vi "FetchRX.vi"(8 "error in (no error)":errorcluster, 11 "reference in":refnum<class "niMmWave_Transceiver.lvclass">) -> (0 "error out":errorcluster, 2 "RX burst data":refnum<class "mmWave data.lvclass">, 3 "reference out":refnum<class "niMmWave_Transceiver.lvclass">)   [LabVIEW 2019, in "niMmWave_Transceiver.lvclass"]
doc: "Fetches RX IQ data from isnturment"
uses:
  niMmWave_Transceiver.lvclass
  C:/Barkhausen mmWave radar/Development/modules/mmw_instrument/src_LabVIEW/Host/SubVIs/mmWave instrument_class/mmWave instrument.lvclass
  mmWave data_class/mmWave data.lvclass
  mmWave HW Control/HW custom error.ctl
  IQBurst_memo_class/IQBurst_memo.lvclass
  C:/Barkhausen mmWave radar/Development/modules/mmw_instrument/src_LabVIEW/Host/SubVIs/mmWave data_class/mmWave data.lvclass
  mmWave instrument_class/Instrument state.ctl
  032ac389-5447-437e-ad81-02506a350dfa.vi
  <vilib>/addons/Modulation/Analog/MT Resample (Complex Cluster).vi
  <vilib>/addons/Modulation/Analog/support/Validators/mod_Fractional Resample Validate.vi
  <vilib>/addons/Modulation/Analog/support/Validators/mod_Check Flush State.vi
  <vilib>/addons/Modulation/Analog/support/mod_FractionalResampler.vi
  <vilib>/addons/Modulation/Analog/support/mod_Integer Rate Interpolation.vi
  <vilib>/addons/Modulation/Analog/support/mod_Set Error Source.vi
  <vilib>/addons/Modulation/Analog/support/Validators/mod_Validate Complex Waveform.vi
  <vilib>/addons/Modulation/Analog/support/mod_PerformResampling.vi
  <vilib>/addons/Modulation/Analog/support/Validators/mod_WFErrorHandler.vi
  <userlib>/_OpenG.lib/string/string.llb/Trim Whitespace (String)__ogtk.vi
  <vilib>/Utility/error.llb/Error Cluster From Error Code.vi
  <vilib>/addons/Modulation/Analog/support/mod_Resampling Factors.vi
  <vilib>/addons/Modulation/Analog/support/mod_ResamplingFilter.vi
  <vilib>/addons/Modulation/Analog/support/mod_Generate Integer Interpolation Filter.vi
  mmWave HW Control/mmWave HW Control.lvlib
  mmWave instrument_class/mmWave instrument.lvclass
panel:
  out "size in":i32
  out "size out":i32
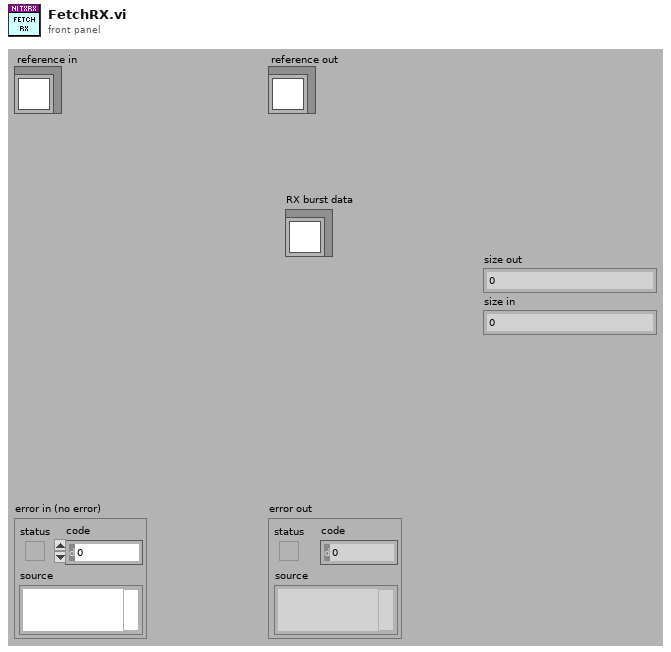
[diagram p1: front panel]
types:
  T1 = typedef "mmWave instrument.lvclass/Instrument state.ctl" = enum16{"Off", "Initialization", "Configuration", "Running", "Calibration"}
  T2 = typedef "mmWave HW Control.lvlib/HW custom error.ctl" = u16
  T3 = typedef "niMmWave_Transceiver.lvclass/ObjectAttributesRef.ctl" = refnum<data-value>
  T4 = typedef "niMmWave_Transceiver.lvclass/ObjectAttributes.ctl" = cluster{"session":T5[], "HW.RX resources":T19, "RF config":T20, "RX trigger options":T21, "TX trigger options":T21, "RX samples":i32, "Downloaded Bursts":map{string, T24}, "TX Fs":dbl, "RX Fs":dbl, "burst sequence":string[]}
  T5 = typedef "Session.ctl" = cluster{"3620 session":refnum<queue>, "tx baseband session":T6, "rx baseband session":T14, "tx gain (dB)":dbl, "rx gain (dB)":dbl, "hardware configuration":T15, "gain ranging":T17[], "pxi trigger bus information":T18}
  T6 = typedef "Tx Baseband Session.ctl" = cluster{"3610 session":T7, "7902 reference":T13}
  T7 = typedef "ni3610_and_ni3630_Driver_Lib.lvlib/Main Settings.ctl" = cluster{"VISA resource name":refnum<visa-resource-name>, "Address Space":T8, "window_offset":u32, "register_addresses":T9, "required_MM_fpga_version":cluster{"signature":u32, "hardware":u32, "current revision":u32, "oldest revision":u32}, "CPLD Oldest Compat Version ":cluster{"hardware":u32, "CPLD firmware":u32}, "MM_FPGA_image_location":string, "is_init":bool, "card_type":T10, "DacLmkConfigFileName":string, "AdcLmkConfigFileName":string, "AdcConfigFileName":string, "DacConfigFileName_RevA":string, "DacConfigFileName_RevB":string, "Mulde hardware revision":u8, "bypass DAC PLL\n":bool, "IQ Card Revision":T11, "board capability":T12}
  T8 = typedef "VISA Register Access Address Space.ctl" = u16
  T9 = typedef "ni3610_and_ni3630_Driver_Lib.lvlib/Register Adresses.ctl" = cluster{"MM based Registers":cluster{"Revision":u32, "OldestCompatRev":u32, "signature":u32, "scratch":u32, "LedControl":u32, "BoardHwRev":u32, "BoardControl":u32, "ThermalStatus":u32, "BasebandStatus":u32, "BasebandControl":u32, "BasebandAuxSetup":u32, "BasebandAuxStatus":u32, "LmkSyncOutSetup":u32, " AdcSyncOutSetup":u32, " InjSyncOutSetup":u32, " PxiTrig0OutSetup":u32, " PxiTrig1OutSetup":u32, " PxiTrig2OutSetup":u32, " PxiTrig3OutSetup":u32, " PxiTrig4OutSetup":u32, " PxiTrig5OutSetup":u32, " PxiTrig6OutSetup":u32, " PxiTrig7OutSetup":u32}, "CPLD based Registers":cluster{"SlaveSignature":u32, "SlaveRevision":u32, "SlaveOldestCompatRev":u32, "SlaveScratch":u32, "SlaveSetup":u32, "SlaveStatus":u32, "IDacReg_offset":u32, "LMKRegGrp0_offset":u32, "QDacReg_offset":u32, "BrdTempSensorVal":u32, "TempSensorPowerDown":u32, "GPIOReg_offset":u32, "IAdcReg_offset":u32, "QAdcReg_offset":u32, "LMKRegGrp1_offset":u32, "QadcTempSensorVal":u32, "IadcTempSensorVal":u32, "RevisionReg":u32, "VcxoReg":u32, "CpldStatusReg":u32, "PowerReg":u32, "VBiasEnReg":u32, "ExtRefOeReg":u32, "QdacCtrlReg":u32, "QdacStatusReg":u32, "IdacCtrlReg":u32, "IdacStatusReg":u32, "QdacJtagIn":u32, "QdacJtagOut":u32, "IdacJtagIn":u32, "IdacJtagOut":u32, "IqDcSetupReg":u32, "QadcStatusReg":u32, "IadcStatusReg":u32, "BrdSetupReg":u32, "IqDcRevisionReg":u32, "PllStatusReg":u32, "EndpointScratchReg":u32, "AdcSyncCfgReg":u32, "IqCardOpampReg":u32}, "CPLD Register Offset":u32, "MM  Register Offset":u32, " PxiTrig0OutSetup":u32}
  T10 = typedef "ni3610_and_ni3630_Driver_Lib.lvlib/Base Card Type.ctl" = enum16{"unspecified", "ADC", "DAC"}
  T11 = typedef "ni3610_and_ni3630_Driver_Lib.lvlib/IQ Card Revision.ctl" = enum16{"RevA", "RevB", "RevC", "RevD"}
  T12 = typedef "ni3610_and_ni3630_Driver_Lib.lvlib/Board Capability.ctl" = cluster{"baseband sync":enum16{"no baseband sync", "baseband sync"}}
  T13 = typedef "Blank FPGA Reference.ctl" = refnum<k20>
  T14 = typedef "Rx Baseband Session.ctl" = cluster{"3630 session":T7, "7902 reference":T13}
  T15 = typedef "Hardware Configuration.ctl" = cluster{"direction":T16, "baseband only":bool}
  T16 = typedef "Direction.ctl" = enum16{"Transceiver", "Receiver", "Transmitter"}
  T17 = typedef "Gain Ranging.ctl" = cluster{"gain ranging active scope":string, "gain ranging stream session":refnum<k20>}
  T18 = typedef "PXI Trigger Bus Info.ctl" = cluster{"chassis resource name":refnum<visa-resource-name>, "7902R (TX)":i16, "3610 (TX)":i16, "3620 (IF)":i16, "3630 (RX)":i16, "7902R (RX)":i16}
  T19 = typedef "mmWave HW Control.lvlib/HW TXRX resources cluster.ctl" = cluster{"TX_DAC":refnum<visa-resource-name>, "TX_FPGA":tag, "IF":tag, "RX_ADC":refnum<visa-resource-name>, "RX_FPGA":tag}
  T20 = typedef "mmWave HW Control.lvlib/HW TXRX RF config cluster.ctl" = cluster{"TX.Frequency":dbl, "TX.Gain":dbl, "TX.mmWave adapter":string, "RX.Frequency":dbl, "RX.Gain":dbl, "RX.mmWave adapter":string}
  T21 = typedef "TX trigger config.ctl" = cluster{"delay":dbl, "trig source":T22, "PXI src":i32, "export":T23, "PXI dest":i32}
  T22 = typedef "FPGA Utility.lvlib/FPGA driver trigger source.ctl" = enum16{"Use Tclk", "PXI_Trig", "Aurora RX trig"}
  T23 = typedef "FPGA Utility.lvlib/FPGA driver trigger destination.ctl" = enum16{"None", "Source trig", "Synced trig", "Delayed sync"}
  T24 = typedef "niMmWave_Transceiver.lvclass/BurstInfo.ctl" = cluster{"starting addr":u32, "end addr":u32}
  T25 = typedef "Constants.ctl" = cluster{"data clock rate (Hz)":dbl, "sample rate (Hz)":dbl, "sample rate selector string":string, "default tx bitfile path":path, "default rx bitfile path":path, "default proc bitfile path":path}
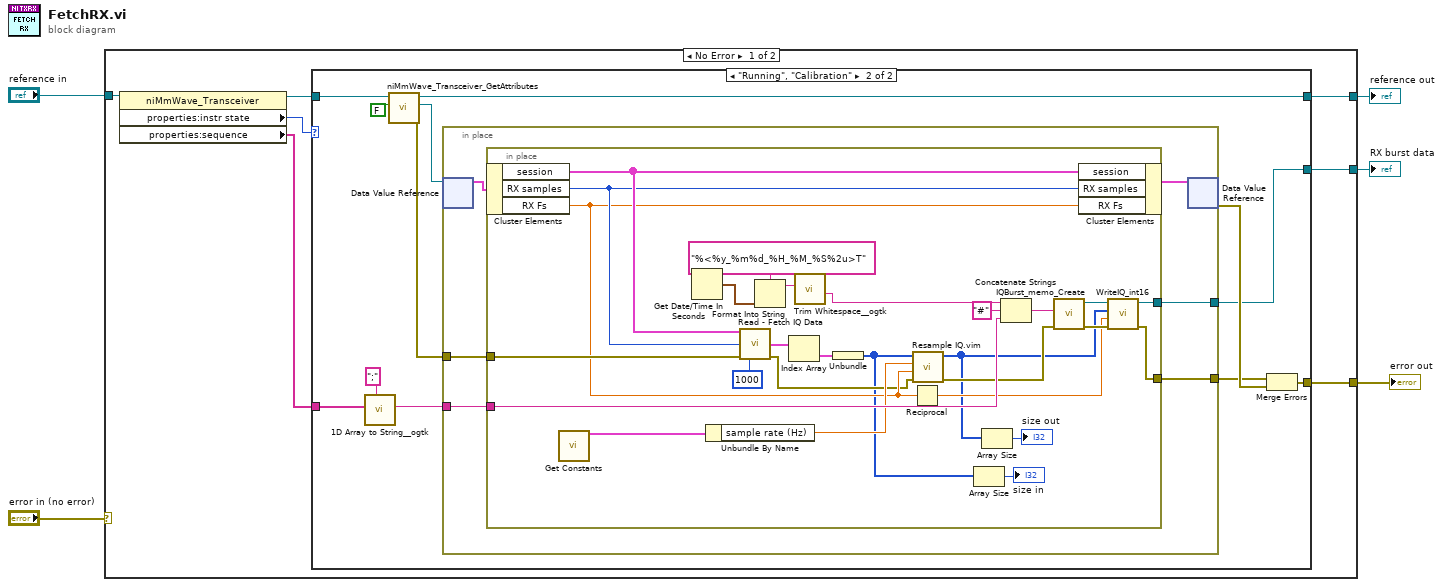
[diagram p0: block diagram]
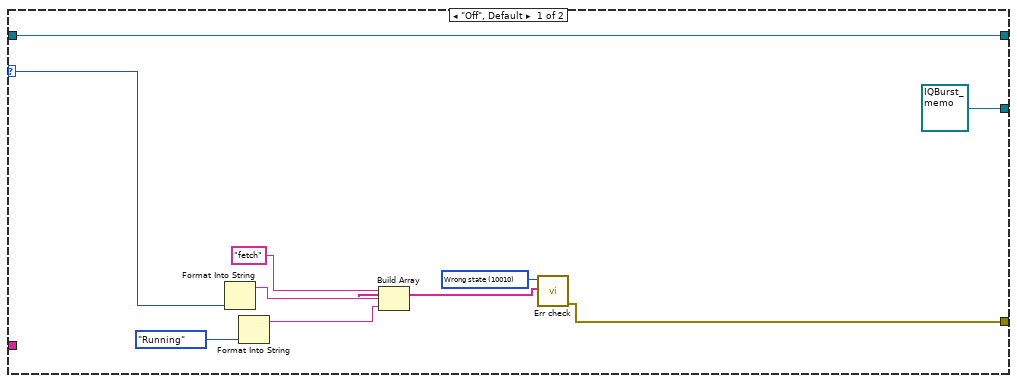
[diagram p2: hidden frame]
diagram:
  n1 = case shown="No Error" "error in (no error)" {
    selector: "error in (no error)" -> [_ w69]
    tunnel: [w12 w69] -> w4
    tunnel: [w11 w68] -> w2
    tunnel: "reference in" -> [w10 w68]
    tunnel: [w7 _] -> w1
    frame No Error {
      n2 = property class="niMmWave_Transceiver"(reference=w10) -> (reference out=w9:refnum<class "niMmWave_Transceiver.lvclass">, "properties:instr state"=w8:T1, "properties:sequence"=w6:string[])  [unwired: 1 in, 1 out]
      n3 = case shown="\"Running\", \"Calibration\"" w8 {
        selector: w8 -> [w19 _]
        tunnel: [w16 w34] -> w12
        tunnel: [w22 w31] -> w11
        tunnel: w9 -> [w22 w29]
        tunnel: [refnum<class "IQBurst_memo.lvclass"> refnum ("reference out") w26] -> w7
        tunnel: w6 -> [_ w27]
        frame "Off", Default {
          w21 = T2 10010 items=["TX list"=10000, "TX length"=10001, "RX length"=10002, "Fs"=10003, "RF Fc"=10004, "Wrong state"=10010] ("HW custom err")
          n4 = Format Into String(w19) -> (resulting string=w18:string)  [unwired: 3 in, 1 out]
          n5 = Format Into String(Instrument_state."Running" ("properties:instr state")) -> (resulting string=w13:string)  [unwired: 3 in, 1 out]
          n6 = Build Array("fetch", w18, w13) -> (w17:string[])
          n7 = call "Err check.vi"("Variant Control"=w17, "HW custom err"=w21) -> ("error out"=w16:errorcluster)  [unwired: 9 in]
        }
        frame "Running", "Calibration" {
          n8 = call <userlib>:"1D Array to String__ogtk.vi"("delimiter (Tab)"=";", "Array of Strings"=w27) -> ("delimited string"=w24:string)  [unwired: 9 in]
          n9 = call "niMmWave_Transceiver_GetAttributes.vi"("return data? (T)"=FALSE, "reference in"=w29) -> ("error out"=w28:errorcluster, "attributes ref"=w30:T3, "reference out"=w31:refnum<class "niMmWave_Transceiver.lvclass">)  [unwired: 6 in, 1 out]
          n10 = in-place {
            in-place-border: w28 -> [w38]
            in-place-border: w24 -> [w37]
            in-place-border: [w36] -> w26
            in-place-border: [w35] -> w25
            n11 = in-place-dvr #1(w30) -> (w39:T4)  [unwired: 1 out]
            n12 = in-place {
              in-place-border: w38 -> [w64]
              in-place-border: w37 -> [w55]
              in-place-border: [w51] -> w36
              in-place-border: [w45] -> w35
              n13 = in-place-cluster #2(w39) -> ("session"=w66:T5[], "RX samples"=w65:i32, "RX Fs"=w49:dbl)
              n14 = call "Get Constants.vi"() -> ("constants"=w58:T25)  [unwired: 15 in]
              n15 = Get Date/Time In Seconds() -> (seconds since 1Jan1904=w61:timestamp)
              n16 = Unbundle By Name(w58) -> ("sample rate (Hz)"=w50:dbl)
              n17 = call "Read - Fetch IQ Data.vi"("session in"=w66, "number of samples"=w65, "error in"=w64, "Timeout (ms)"=1000) -> ("data [channel]"=w63:cluster{"data":i16[]}[], "error out"=w47:errorcluster)  [unwired: 9 in, 1 out]
              n18 = Format Into String(format string="%<%y_%m%d_%H_%M_%S%2u>T", w61) -> (resulting string=w59:string)  [unwired: 2 in, 1 out]
              n19 = Index Array(array=w63) -> (element=w62:cluster{"data":i16[]})  [unwired: 1 in]
              n20 = call-poly <userlib>:"Trim Whitespace__ogtk.vi"("String in"=w59) -> ("String out"=w57:string)  [unwired: 6 in]
              n21 = Unbundle(w62) -> ("data"=w44:i16[])
              n22 = Reciprocal(x=w49) -> (1/x=w48:dbl)
              n23 = call "Resample IQ.vim"("error in (no error)"=w47, "FS out"=w49, "Fs in"=w50, "data in"=w44) -> ("error out"=w46:errorcluster, "resampled data"=w43:i16[])  [unwired: 6 in]
              n24 = Array Size(array=w44) -> (size(s)=→"size in":i32)
              n25 = Array Size(array=w43) -> (size(s)=→"size out":i32)
              n26 = Concatenate Strings(w57, "#" ("string"), w55) -> (w54:string)
              n27 = call "IQBurst_memo_Create.vi"("error in (no error)"=w46, "burst name"=w54) -> ("error out"=w53:errorcluster, "reference out"=w52:refnum<class "IQBurst_memo.lvclass">)  [unwired: 8 in]
              n28 = in-place-cluster #2("session"=w66, "RX samples"=w65, "RX Fs"=w49) -> (w40:T4)
              n29 = call-dynamic "WriteIQ_int16.vi"("error in (no error)"=w53, "dt"=w48, "data"=w43, "reference in"=w52) -> ("error out"=w45:errorcluster, "reference out"=w51:refnum<class "IQBurst_memo.lvclass">)  [unwired: 6 in]
            }
            n30 = in-place-dvr #1(w40) -> (w33:errorcluster)  [unwired: 1 out]
          }
          n31 = Merge Errors(w25, w33) -> (w34:errorcluster)
        }
      }
    }
    frame Error {
    }
  }
  "error out" <- w4
  "reference out" <- w2
  "RX burst data" <- w1
